vi "MdfClose.vi"(8 "error in (no error)":errorcluster, 11 "MDFRef":refnum<k24>) -> (0 "error IO":errorcluster)   [LabVIEW 2025, in "MdfFile.lvlib"]
uses:
  MdfFile.lvlib
  data/mdflibrary.dll
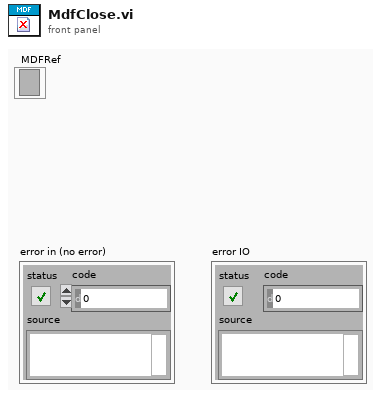
[diagram p1: front panel]
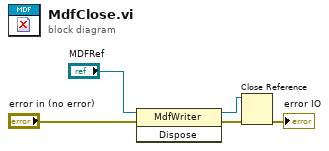
[diagram p0: block diagram]
diagram:
  n1 = invoke class="MdfWriter" method="Dispose"(reference="MDFRef", error in="error in (no error)") -> (reference out=w3:refnum<k24>, error out=w2:errorcluster)  [unwired: 1 in, 1 out]
  n2 = Close Reference(reference=w3, error in (no error)=w2) -> (error out=→"error IO":errorcluster)
